vi "To and From CSV Test.vi"() -> (0 "error out":errorcluster, 1 "Pass":bool, 2 "Lines Equal":bool, 3 "Class Equal":bool)   [LabVIEW 2015, in "Increment tests.lvlib"]
uses:
  Increment tests.lvlib
  <vilib>/NI/Module Execution Interface/Engine Configuration/engine configuration.lvclass
  editor node/Increment editor node.lvclass
  module/configuration/Increment configuration.lvclass
  module/configuration/Increment configuration.lvclass/Increment configuration.ctl
  <vilib>/NI/Configuration Framework/serializable configuration/NISE_CEF_serializable configuration.lvclass/NISE_CEF_serializable configuration.ctl
  <vilib>/Utility/LVClass/Get LV Class Name.vi
  <vilib>/NI/Configuration Framework/error generator/NISE_error generator.vi
  <vilib>/NI/Tag Bus Module Framework/channel/TBM channel.lvclass
  <vilib>/NI/Configuration Framework/serializable configuration/NISE_CEF_serializable configuration.lvclass
panel:
  out "Write Channels":bool
  out "Read Channels":bool
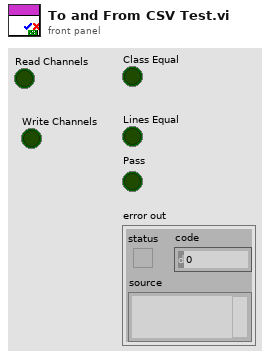
[diagram p1: front panel]
types:
  T1 = typedef "Increment configuration.lvclass/Line.ctl" = cluster{"Name":string, "channel in":refnum<class "TBM channel.lvclass">, "channel out":refnum<class "TBM channel.lvclass">}
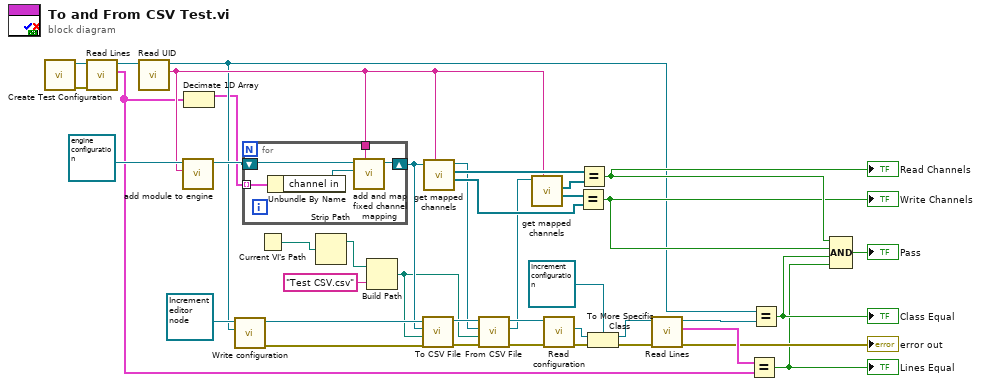
[diagram p0: block diagram]
diagram:
  n1 = call "Create Test Configuration.vi"() -> ("error out"=w39:errorcluster, "Module Configuration"=w40:refnum<class "Increment configuration.lvclass">)  [unwired: 6 in, 4 out]
  n2 = call "Read Lines.vi"("error in (no error)"=w39, "Increment configuration in"=w40) -> ("Lines"=w2:T1[], "Increment configuration out"=w27:refnum<class "Increment configuration.lvclass">)  [unwired: 7 in, 1 out]
  n3 = call <vilib>:"Read UID.vi"("configuration in"=w27) -> ("instance id"=w6:string, "configuration out"=w3:refnum<class "Increment configuration.lvclass">)  [unwired: 8 in, 1 out]
  n4 = call-dynamic "add module to engine.vi"("module ID"=w6, "engine configuration in"=refnum<class "engine configuration.lvclass"> refnum ("engine configuration")) -> ("engine configuration out"=w26:refnum<class "engine configuration.lvclass">)  [unwired: 8 in, 1 out]
  n5 = Decimate 1D Array(w2) -> (w1:T1[])  [unwired: 1 out]
  n6 = call-dynamic "Write configuration.vi"("configuration"=w3, "Increment editor node in"=refnum<class "Increment editor node.lvclass"> refnum ("tag bus configurable plugin editor node")) -> ("error out"=w20:errorcluster, "Increment editor node out"=w25:refnum<class "Increment editor node.lvclass">)  [unwired: 8 in]
  n7 = for {
    tunnel: w1 -> [w44] mode=indexing
    tunnel: w6 -> [w43]
    shift-right: [w42] -> w18
    shift-left: w26 -> [w41]
    n8 = Unbundle By Name(w44) -> ("channel in"=w45:refnum<class "TBM channel.lvclass">)
    n9 = call <vilib>:"add and map fixed channel mapping.vi"("module instance"=w43, "fixed channel"=w45, "engine configuration in"=w41) -> ("engine configuration out"=w42:refnum<class "engine configuration.lvclass">)  [unwired: 7 in, 1 out]
  }
  n10 = Current VI's Path() -> (path=w15:path)
  n11 = Strip Path(path=w15) -> (stripped path=w14:path)  [unwired: 1 out]
  n12 = Build Path(base path=w14, name or relative path="Test CSV.csv") -> (appended path=w13:path)
  n13 = call-dynamic "To CSV File.vi"("error in (no error)"=w20, "Path"=w13, "engine configuration"=w18, "Increment editor node in"=w25) -> ("error out"=w21:errorcluster, "Increment editor node out"=w23:refnum<class "Increment editor node.lvclass">)  [unwired: 6 in]
  n14 = call-dynamic "get mapped channels.vi"("owner"=w6, "engine configuration in"=w18) -> ("write channels"=w31:refnum<class "TBM channel.lvclass">[], "read channels"=w33:refnum<class "TBM channel.lvclass">[], "engine configuration out"=w17:refnum<class "engine configuration.lvclass">)  [unwired: 5 in, 2 out]
  n15 = call-dynamic "From CSV File.vi"("error in (no error)"=w21, "Path"=w13, "engine in"=w17, "Increment editor node in"=w23) -> ("error out"=w22:errorcluster, "engine out"=w12:refnum<class "engine configuration.lvclass">, "Increment editor node out"=w24:refnum<class "Increment editor node.lvclass">)  [unwired: 4 in, 1 out]
  n16 = call-dynamic "get mapped channels.vi"("owner"=w6, "engine configuration in"=w12) -> ("write channels"=w32:refnum<class "TBM channel.lvclass">[], "read channels"=w34:refnum<class "TBM channel.lvclass">[])  [unwired: 5 in, 3 out]
  n17 = call-dynamic "Read configuration.vi"("error in"=w22, "Increment editor node in"=w24) -> ("error out"=w8:errorcluster, "configuration"=w9:refnum<class "NISE_CEF_serializable configuration.lvclass">)  [unwired: 7 in, 1 out]
  n18 = Equal?(x=w32, y=w31) -> (x = y?=w28:bool)
  "Write Channels" <- w28
  n19 = Equal?(x=w33, y=w34) -> (x = y?=w29:bool)
  "Read Channels" <- w29
  n20 = To More Specific Class(target class=refnum<class "Increment configuration.lvclass"> refnum ("tag bus configurable plugin module configuration"), reference=w9, error in=w8) -> (specific class reference=w10:refnum<class "Increment configuration.lvclass">, error out=w7:errorcluster)
  n21 = call "Read Lines.vi"("error in (no error)"=w7, "Increment configuration in"=w10) -> ("error out"=→"error out":errorcluster, "Lines"=w37:T1[], "Increment configuration out"=w38:refnum<class "Increment configuration.lvclass">)  [unwired: 7 in]
  n22 = Equal?(x=w37, y=w2) -> (x = y?=w4:bool)
  "Lines Equal" <- w4
  n23 = Equal?(x=w3, y=w38) -> (x = y?=w5:bool)
  "Class Equal" <- w5
  n24 = Compound Arithmetic op=AND(w29, w28, w5, w4) -> (→"Pass":bool)
